vi "Convert XNET Table Attribute to VS Table.vi"(11 "attribute text":string) -> (1 "Value":i64[](array[numeric]), 2 "Names":string[](array[string]))   [LabVIEW 2025, in "Protection and Counter Addon System Explorer.lvlib"]
uses:
  Protection and Counter Addon System Explorer.lvlib
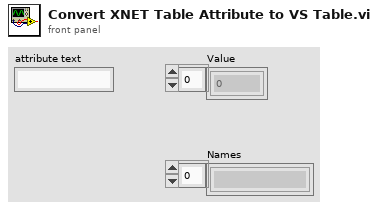
[diagram p1: front panel]
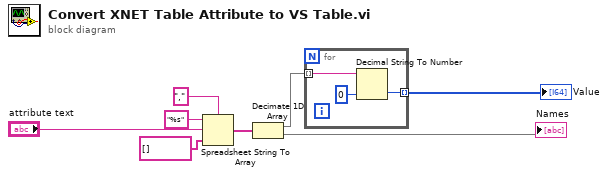
[diagram p0: block diagram]
diagram:
  n1 = Spreadsheet String To Array(delimiter (Tab)=",", format string="%s", spreadsheet string="attribute text", array type (2D Dbl)=string[] []) -> (array=w5:string[])
  n2 = Decimate 1D Array(w5) -> (w6:string[], →"Names":string[])
  n3 = for {
    tunnel: w6 -> [w11] mode=indexing
    tunnel: [w9] -> w7 mode=indexing
    n4 = Decimal String To Number(string=w11, default (0L)=i64 0 ("default (0 I32)")) -> (number=w9:i64)  [unwired: 1 in, 1 out]
  }
  "Value" <- w7
